vi "340 Read and Compressor auto control(SubVI).vi"(11 "Instrument":T2={"limit"={"Field limit"=0.0, "Field rate limit"=0.0, "Temp limit"=0.0, "Temp low limit"=0.0, "Temp rate limit "=0.0}, "genarl"={"行数"=refnum, "编辑列表框？"=refnum, "列表框"=refnum, "camg 振荡状态"=refnum, "Aborting"=refnum, "数据文件"=refnum, "warning"=refnum, "vi路径"="", "Instrument Type"=enum."PPMS-Rotate"}, "cmag"={"TM620"="TCPIP0::192.168.1.5::4266::SOCKET", "M24C Resource"="GPIB0::24::INSTR", "4G supply"="", "Temp Status 24C"=refnum, "Temp"=refnum, "9T信号"=refnum, "4g supply status"=refnum, "in-plane"="", "out-plane"="", "in-plane signal"=FALSE, "out-plane signal"=FALSE, "in plane 信号"=refnum, "pzt volt"=refnum, "camg Rate"=refnum}, "lengtou2"={"750 visa"="", "750 rotate"="", "semaphore 340"=refnum, "semaphore 750"=refnum, "750 field status"=refnum, "Input (0:A) 340"=0, "340 Resource"="GPIB0::14::INSTR", "340 Status"=refnum, "Input (0:B) 340"=1, "Loop (0: 1)"=0, "Loop (1: 1)"=0, "TCP master instance"=refnum}, "lengtou"={"TCP master instance"=refnum, "335 Status"=refnum, "335 Resource "="GPIB0::24::INSTR", "Input (0:A) 335"=0, "Input (0:B) 335"=1, "Heater Output (1:1) 335"=1, "semaphore 335"=refnum}, "325 for test"={"quantum design"=refnum, "semaphore 325"=refnum, "325 Resource "="GPIB0::13::INSTR", "Input (0:A) 325"=0, "Heater Output (1:1) 325"=1, "325 Status"=refnum}} {"325 for test"."Heater Output (1:1) 325" items=["1"=1, "2"=2]; "325 for test"."Input (0:A) 325" items=["A", "B"]; "lengtou"."Heater Output (1:1) 335" items=["1"=1, "2"=2]; "lengtou"."Input (0:B) 335" items=["A", "B"]; "lengtou"."Input (0:A) 335" items=["A", "B"]; "lengtou2"."Loop (1: 1)" items=["1", "2"]; "lengtou2"."Loop (0: 1)" items=["1", "2"]; "lengtou2"."Input (0:B) 340" items=["A", "B", "C", "D"]; "lengtou2"."Input (0:A) 340" items=["A", "B", "C", "D"]}) -> (2 "Output Field (Gs)":dbl, 3 "output":T7 {"?" items=["Unknow", "Stable", "Following Warm", "Following Cold", "Unfollowing"]; "?" items=["Unknow", "Stable", "Following Warm", "Following Cold", "Unfollowing"]}, 9 "field status 2":T1=enum."Stable")   [LabVIEW 2019, in "Get value.lvlib"]
uses:
  Get value.lvlib
  ctl/335 state.ctl
  ctl/Instrument.ctl
  <vilib>/NI/Modbus Library/API/Master/Modbus Master.lvclass
  ctl/limit.ctl
  ctl/warning.ctl
  ctl/Instrument Type.ctl
  ctl/9T mag field stauts.ctl
  C:/Users/fuyang/Desktop/postdoctor/labview/labview-measure/lib/QDInstrument.dll
  lib/QDInstrument.dll
  lib/Lake Shore 340/Lake Shore Cryotronics 340.lvlib
  User lib.lvlib
panel:
  out "下拉列表 2":T6=2 items=["Unknow", "Stable", "Following Warm", "Following Cold", "Unfollowing"]
  out "下拉列表":T6=2 items=["Unknow", "Stable", "Following Warm", "Following Cold", "Unfollowing"]
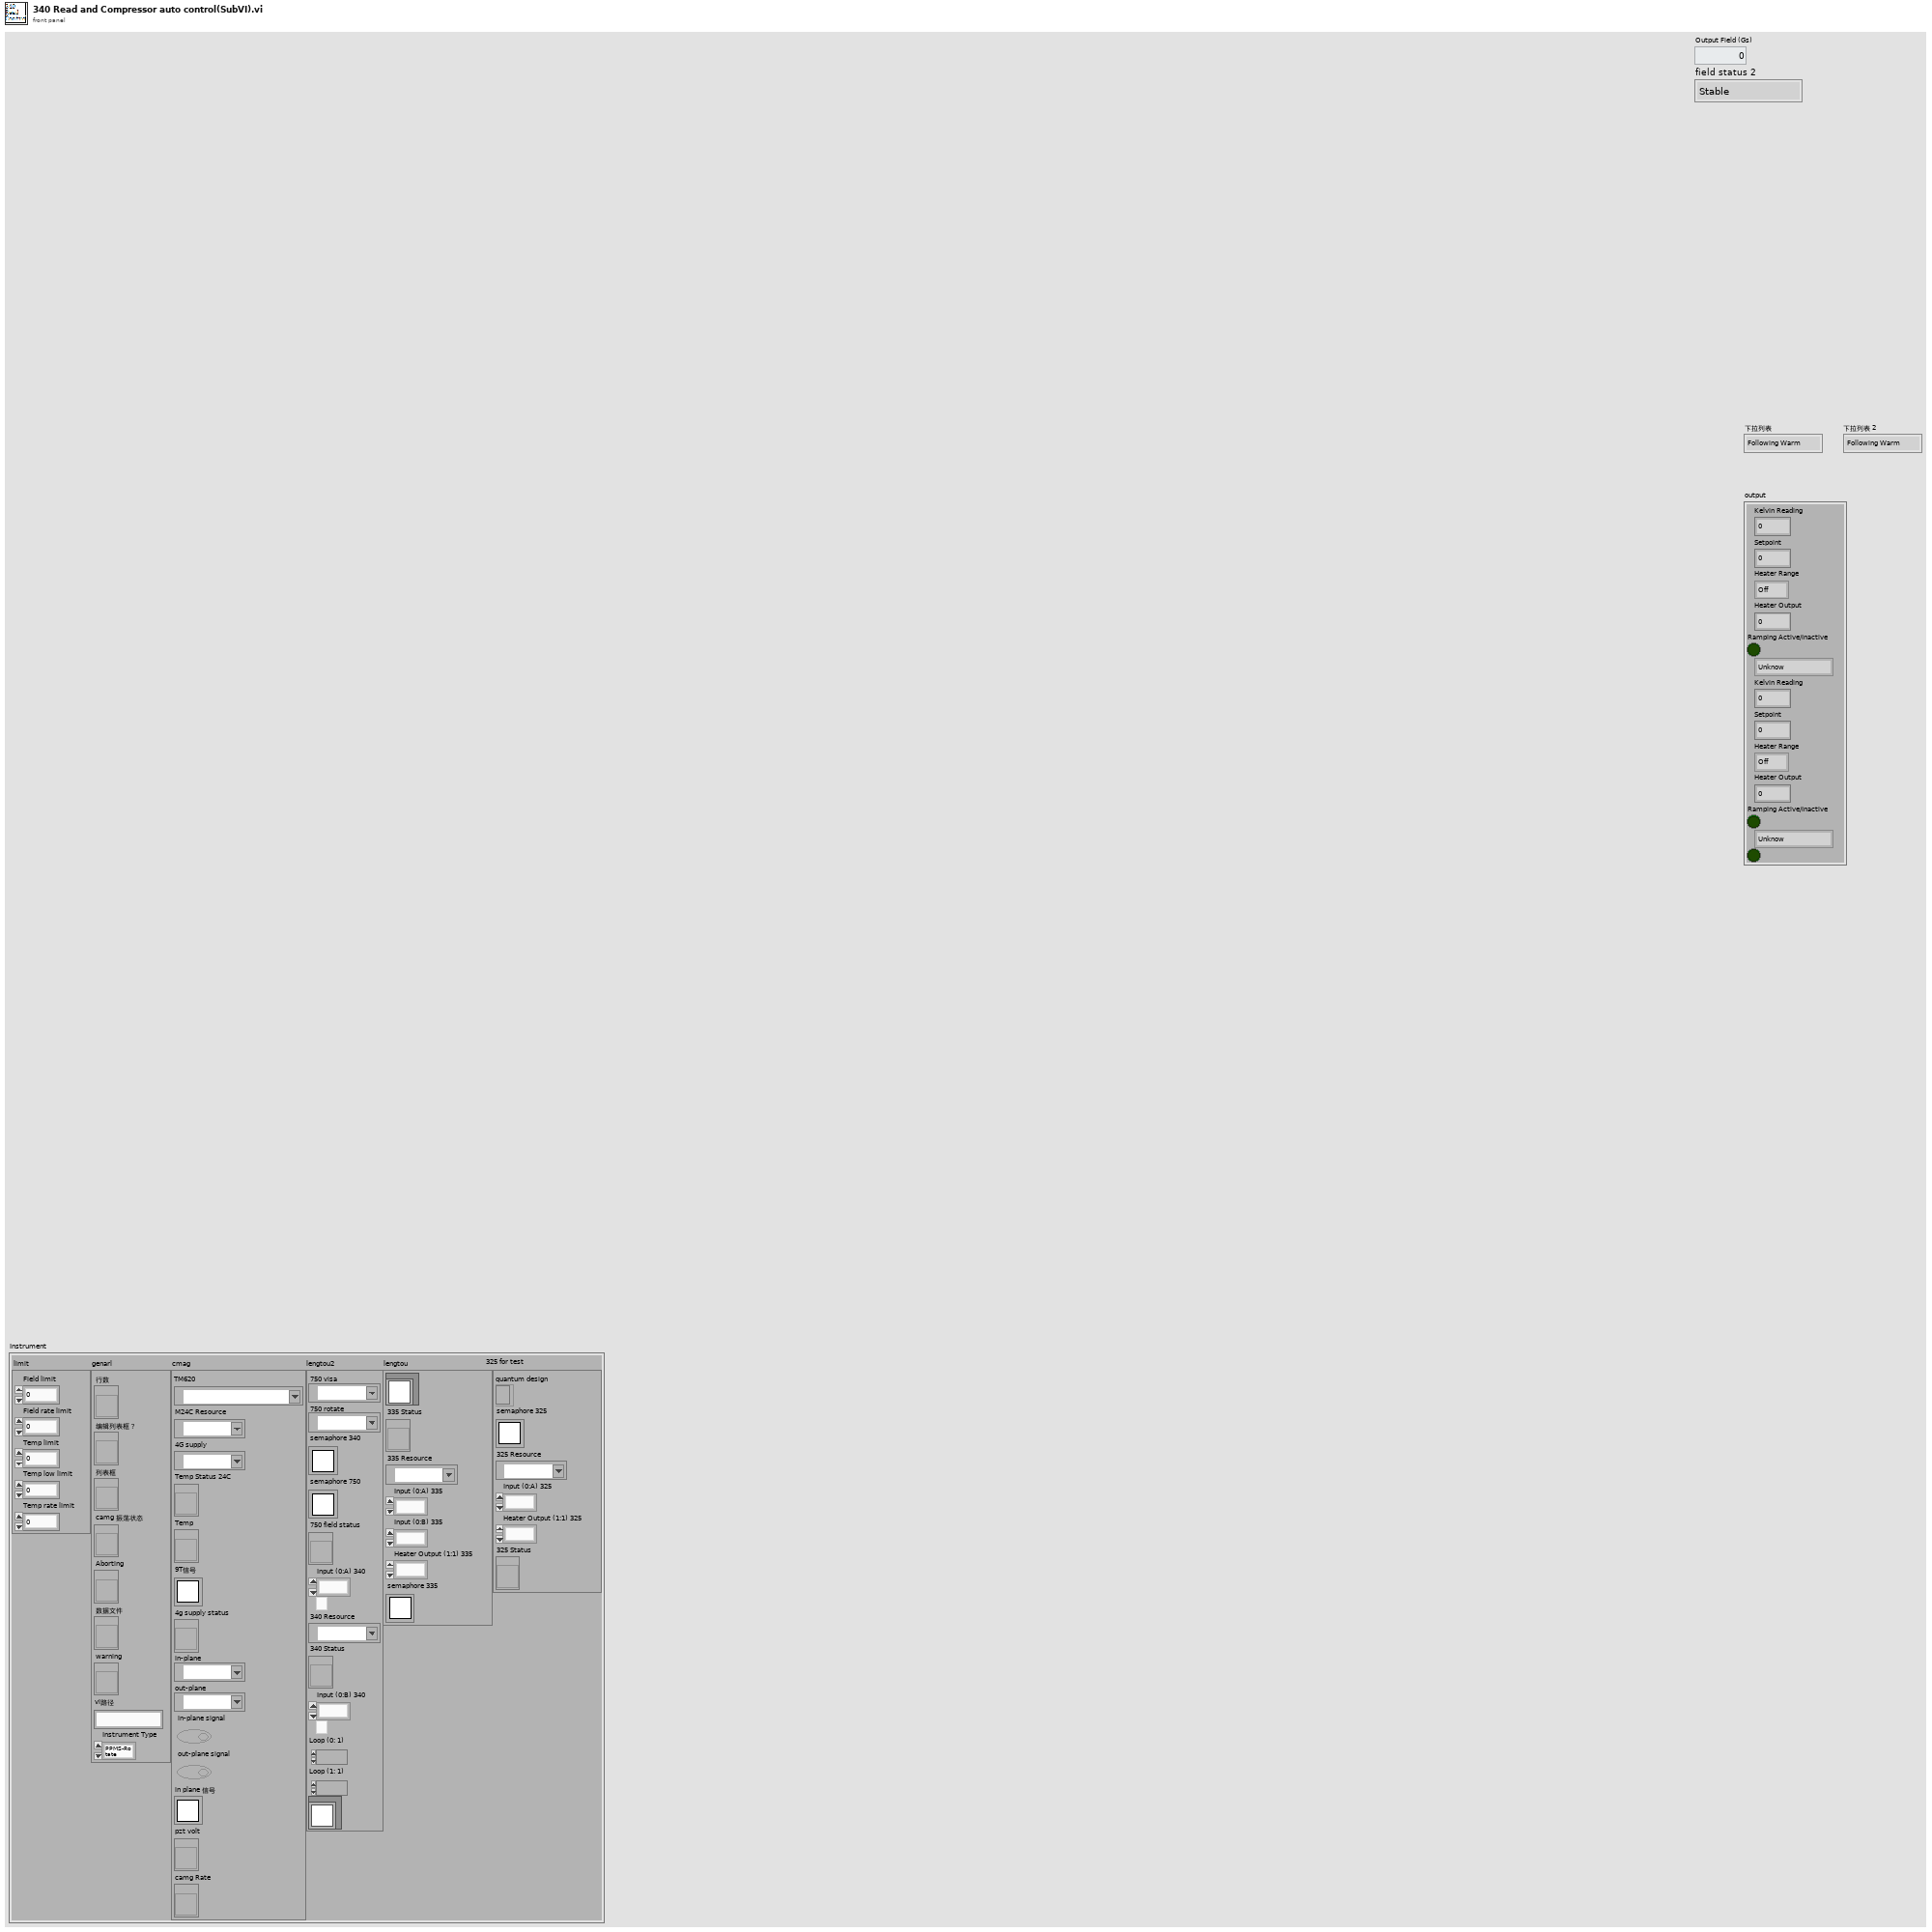
[diagram p1: front panel]
types:
  T1 = typedef "9T mag field stauts.ctl" = enum16{"unknow", "Stable", "Sweep up", "Sweep down", "Sweep to zero", "Pause"}
  T2 = typedef "Instrument.ctl" = cluster{"limit":T3, "genarl":cluster{"行数":refnum<vi>, "编辑列表框？":refnum<vi>, "列表框":refnum<vi>, "camg 振荡状态":refnum<vi>, "Aborting":refnum<vi>, "数据文件":refnum<vi>, "warning":refnum<vi>, "vi路径":string, "Instrument Type":T4}, "cmag":cluster{"TM620":refnum<visa-resource-name>, "M24C Resource":refnum<visa-resource-name>, "4G supply":refnum<visa-resource-name>, "Temp Status 24C":refnum<vi>, "Temp":refnum<vi>, "9T信号":T5, "4g supply status":refnum<vi>, "in-plane":refnum<visa-resource-name>, "out-plane":refnum<visa-resource-name>, "in-plane signal":bool, "out-plane signal":bool, "in plane 信号":T5, "pzt volt":refnum<vi>, "camg Rate":refnum<vi>}, "lengtou2":cluster{"750 visa":refnum<visa-resource-name>, "750 rotate":refnum<visa-resource-name>, "semaphore 340":T5, "semaphore 750":T5, "750 field status":refnum<vi>, "Input (0:A) 340":u16, "340 Resource":refnum<visa-resource-name>, "340 Status":refnum<vi>, "Input (0:B) 340":u16, "Loop (0: 1)":u16, "Loop (1: 1)":u16, "TCP master instance":refnum<class "Modbus Master.lvclass">}, "lengtou":cluster{"TCP master instance":refnum<class "Modbus Master.lvclass">, "335 Status":refnum<vi>, "335 Resource ":refnum<visa-resource-name>, "Input (0:A) 335":u16, "Input (0:B) 335":u16, "Heater Output (1:1) 335":u16, "semaphore 335":T5}, "325 for test":cluster{"quantum design":refnum<k24>, "semaphore 325":T5, "325 Resource ":refnum<visa-resource-name>, "Input (0:A) 325":u16, "Heater Output (1:1) 325":u16, "325 Status":refnum<vi>}}
  T3 = typedef "limit.ctl" = cluster{"Field limit":dbl, "Field rate limit":dbl, "Temp limit":dbl, "Temp low limit":dbl, "Temp rate limit ":dbl}
  T4 = typedef "Instrument Type.ctl" = enum16{"PPMS", "VersaLab", "DynaCool", "SVSM", "PPMS-Rotate", "Lakeshore335", "2T cmag", "9T mag old", "9T cmag", "9T cmag DAC", "9T cmag rotate", "test"}
  T5 = typedef "Semaphore RefNum" = refnum<k1>
  T6 = typedef "335 state.ctl" = u16
  T7 = cluster{"Kelvin Reading":dbl, "Setpoint":dbl, "Heater Range":enum16{"Off", "1", "2", "3", "4", "5"}, "Heater Output":dbl, "Ramping Active/Inactive":bool, T6, "Kelvin Reading":dbl, "Setpoint":dbl, "Heater Range":enum16{"Off", "1", "2", "3", "4", "5"}, "Heater Output":dbl, "Ramping Active/Inactive":bool, T6, bool}
  T8 = cluster{"Kelvin Reading":dbl, "Setpoint":dbl, "Heater Range 340-Loop2":i32, "Output Value":dbl, "Ramping Active/Inactive":bool, T6, "Kelvin Reading":dbl, "Setpoint":dbl, "Heater Range":enum16{"Off", "1", "2", "3", "4", "5"}, "Heater Output":dbl, "Ramping Active/Inactive":bool, T6, bool}
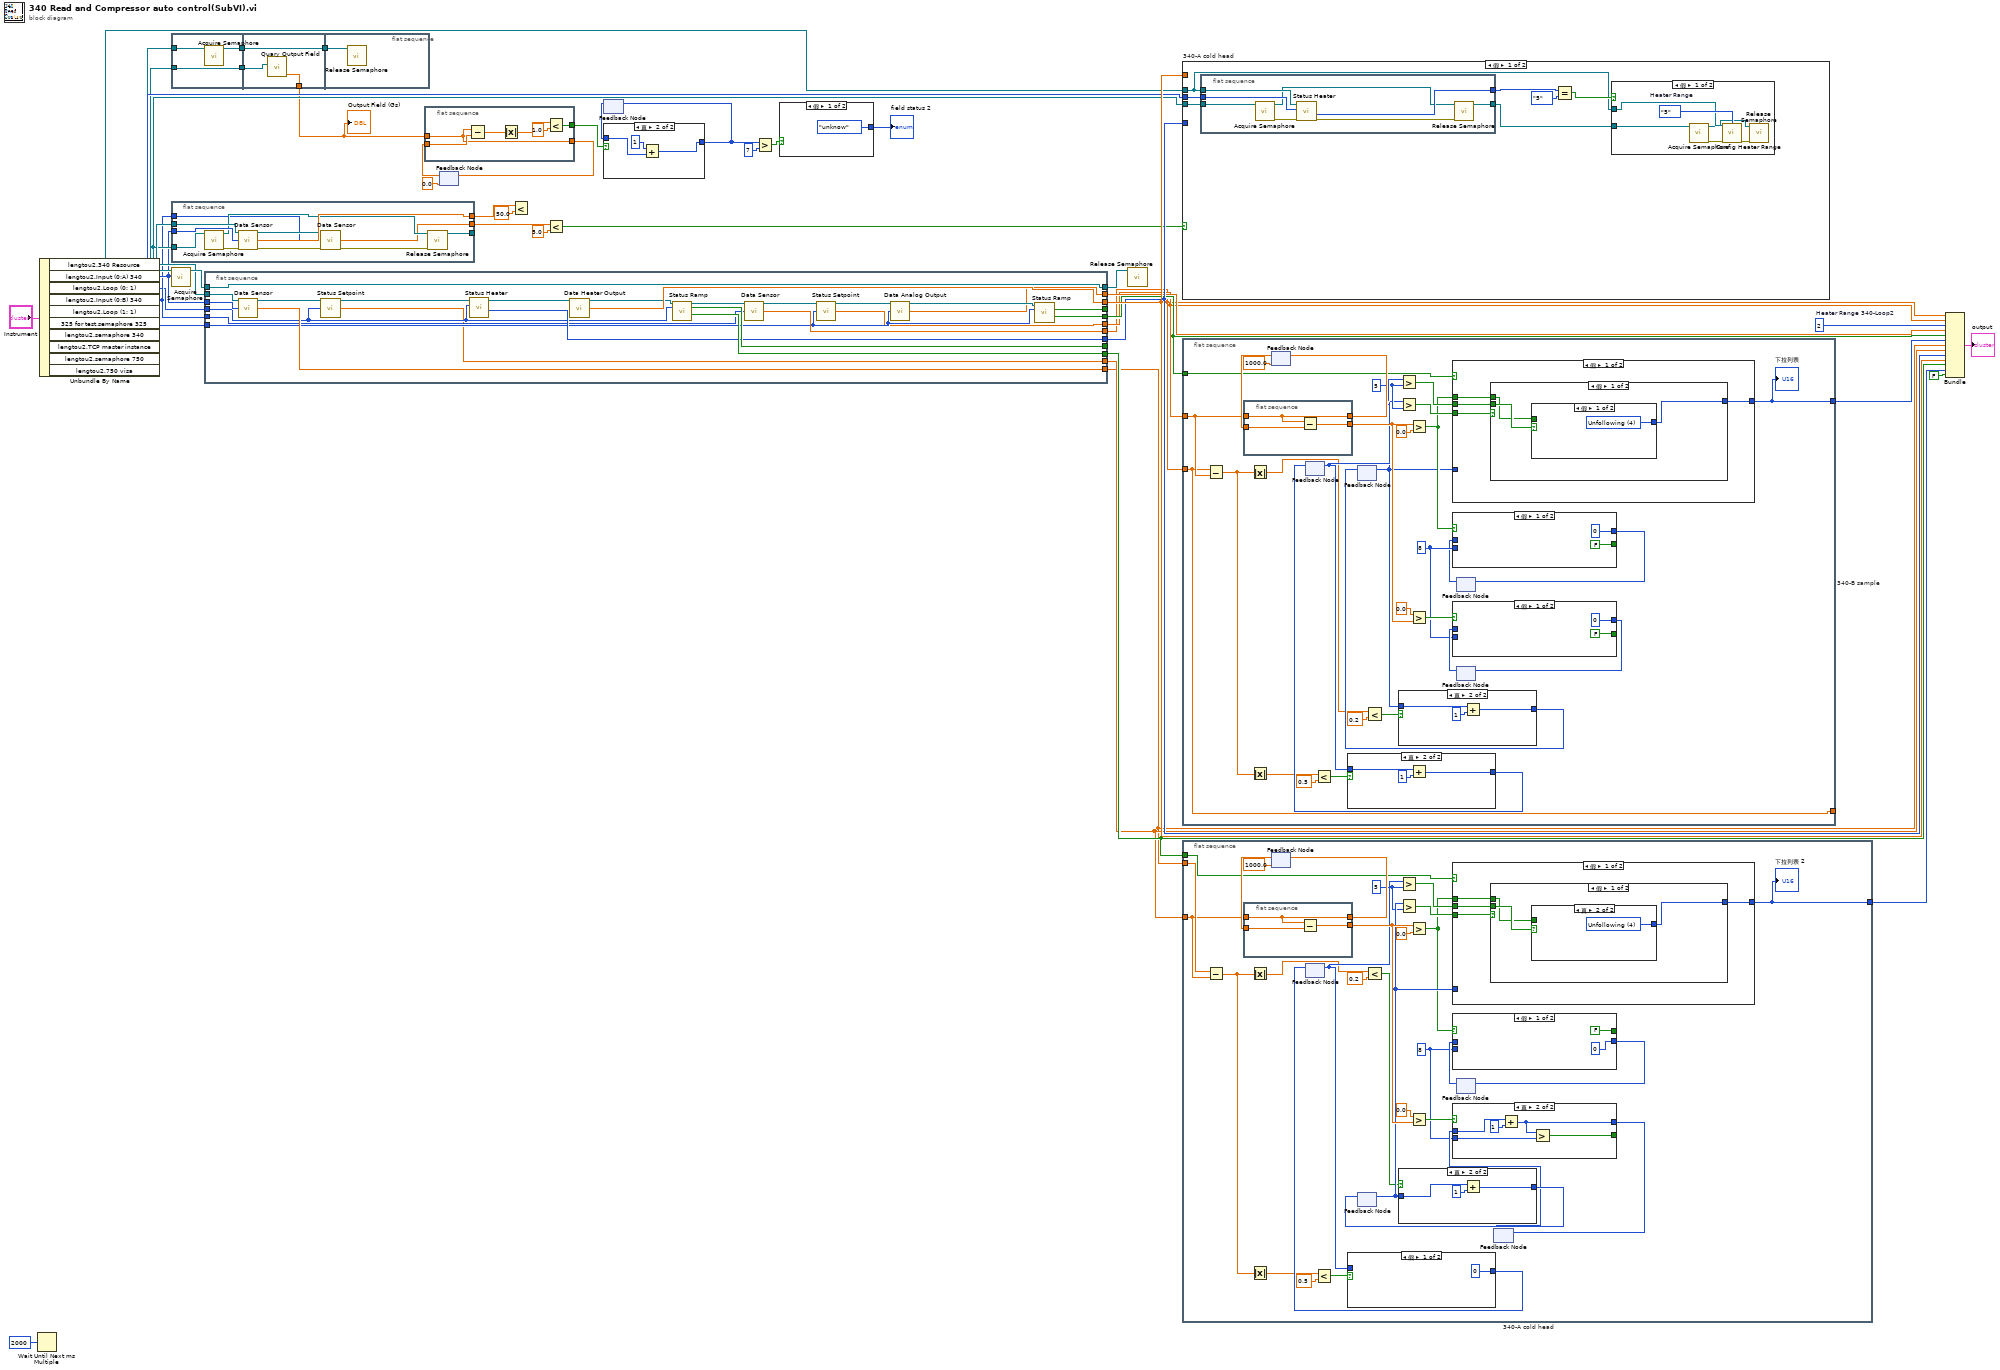
[diagram p0: block diagram]
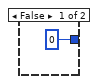
[diagram p2: hidden frame]
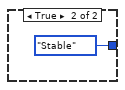
[diagram p3: hidden frame]
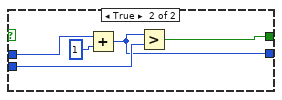
[diagram p4: hidden frame]
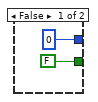
[diagram p5: hidden frame]
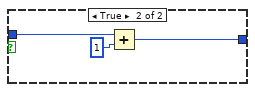
[diagram p6: hidden frame]
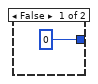
[diagram p7: hidden frame]
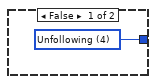
[diagram p8: hidden frame]
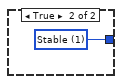
[diagram p9: hidden frame]
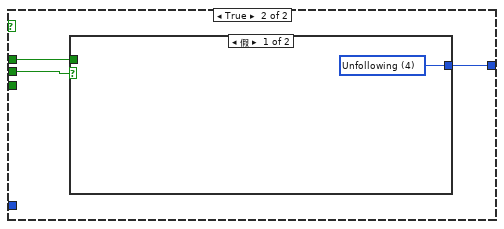
[diagram p10: hidden frame]
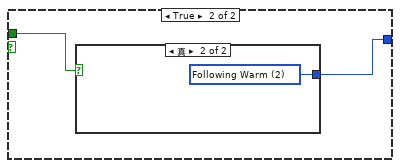
[diagram p11: hidden frame]
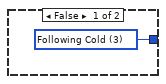
[diagram p12: hidden frame]
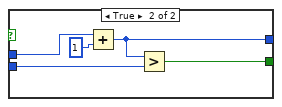
[diagram p13: hidden frame]
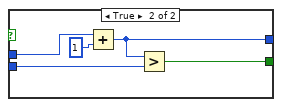
[diagram p14: hidden frame]
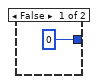
[diagram p15: hidden frame]
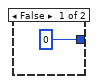
[diagram p16: hidden frame]
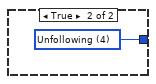
[diagram p17: hidden frame]
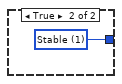
[diagram p18: hidden frame]
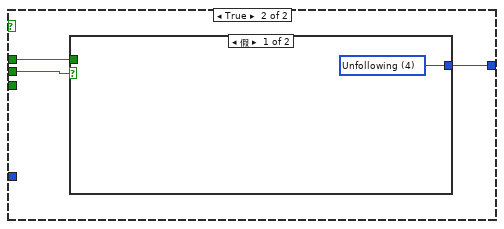
[diagram p19: hidden frame]
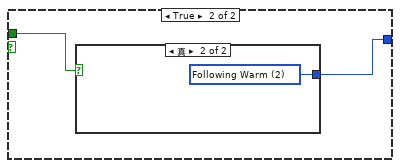
[diagram p20: hidden frame]
diagram:
  w22 = 2  # Heater Range 340-Loop2
  n1 = Wait Until Next ms Multiple(millisecond multiple=u32 2000) -> ()  [unwired: 1 out]
  n2 = Unbundle By Name("Instrument") -> ("lengtou2.340 Resource"=w31:refnum<visa-resource-name>, "lengtou2.Input (0:A) 340"=w28:u16, "lengtou2.Loop (0: 1)"=w24:u16, "lengtou2.Input (0:B) 340"=w27:u16, "lengtou2.Loop (1: 1)"=w23:u16, "lengtou2.semaphore 340"=w29:T5, "lengtou2.semaphore 750"=w17:T5, "lengtou2.750 visa"=w19:refnum<visa-resource-name>)  [unwired: 2 out]
  n3 = flat-sequence {
    tunnel: w19 -> [w47]
    tunnel: [w47] -> w18
    tunnel: w17 -> [w45]
    tunnel: [w46] -> w16
    tunnel: w18 -> [w50]
    tunnel: w16 -> [w49]
    tunnel: [w49] -> w15
    tunnel: [w48] -> w14
    tunnel: w15 -> [w51]
    frame #0 {
      n4 = call <vilib>:"Acquire Semaphore.vi"("semaphore"=w45) -> ("semaphore out"=w46:T5)  [unwired: 4 in, 2 out]
    }
    frame #1 {
      n5 = call "Quary Output Field.vi"("VISA resource name"=w50) -> ("Output Field (Gs)"=w48:dbl)  [unwired: 8 in, 2 out]
    }
    frame #2 {
      n6 = call <vilib>:"Release Semaphore.vi"("semaphore"=w51) -> ()  [unwired: 5 in, 2 out]
    }
  }
  n7 = flat-sequence {
    tunnel: [w63] -> w32
    tunnel: w31 -> [w62]
    tunnel: w28 -> [w61]
    tunnel: w29 -> [w60]
    tunnel: [w57] -> _
    tunnel: w27 -> [w53]
    tunnel: [w52] -> w30
    frame #0 {
      n8 = call <vilib>:"Acquire Semaphore.vi"("semaphore"=w60) -> ("error out"=w59:errorcluster, "semaphore out"=w58:T5)  [unwired: 4 in, 1 out]
      n9 = call "Data Sensor.vi"("VISA resource name"=w62, "Input (0: A)"=w61, "error in (no error)"=w59) -> ("VISA resource name out"=w54:refnum<visa-resource-name>, "Kelvin Reading"=w63:dbl, "error out"=w56:errorcluster)  [unwired: 8 in, 2 out]
      n10 = call "Data Sensor.vi"("VISA resource name"=w54, "Input (0: A)"=w53, "error in (no error)"=w56) -> ("Kelvin Reading"=w52:dbl, "error out"=w55:errorcluster)  [unwired: 8 in, 3 out]
      n11 = call <vilib>:"Release Semaphore.vi"("error in (no error)"=w55, "semaphore"=w58) -> ("semaphore out"=w57:T5)  [unwired: 4 in, 1 out]
    }
  }
  n12 = call <vilib>:"Acquire Semaphore.vi"("semaphore"=w29) -> ("semaphore out"=w42:T5)  [unwired: 4 in, 2 out]
  n13 = flat-sequence {
    tunnel: [w64] -> w4
    tunnel: w31 -> [w87]
    tunnel: w42 -> [w88]
    tunnel: [w88] -> w43
    tunnel: w28 -> [w77]
    tunnel: [w86] -> w37
    tunnel: [w85] -> w2
    tunnel: [w83] -> _
    tunnel: [w82] -> w41
    tunnel: w24 -> [w68]
    tunnel: [w78] -> w38
    tunnel: [w76] -> w1
    tunnel: w27 -> [w74]
    tunnel: [w65] -> w3
    tunnel: [w71] -> w25
    tunnel: [w70] -> _
    tunnel: [w69] -> w26
    tunnel: w23 -> [w67]
    frame #0 {
      n14 = call "Data Sensor.vi"("VISA resource name"=w87, "Input (0: A)"=w77) -> ("VISA resource name out"=w84:refnum<visa-resource-name>, "Kelvin Reading"=w85:dbl)  [unwired: 9 in, 3 out]
      n15 = call "Status Setpoint.vi"("VISA resource name"=w84, "Loop (0: 1)"=w68) -> ("VISA resource name out"=w80:refnum<visa-resource-name>, "Setpoint"=w64:dbl)  [unwired: 11 in, 1 out]
      n16 = call "Status Heater.vi"("Loop"=w68, "VISA resource name"=w80) -> ("Heater Range"=w78:enum16{"Off", "1", "2", "3", "4", "5"}, "VISA resource name out"=w79:refnum<visa-resource-name>)  [unwired: 7 in, 1 out]
      n17 = call "Data Heater Output.vi"("VISA resource name"=w79) -> ("VISA resource name out"=w81:refnum<visa-resource-name>, "Heater Output"=w82:dbl)  [unwired: 12 in, 1 out]
      n18 = call "Status Ramp.vi"("VISA resource name"=w81, "Loop (0: 1)"=w68) -> ("VISA resource name out"=w75:refnum<visa-resource-name>, "Ramping On/Off"=w83:bool, "Ramping Active/Inactive"=w86:bool)  [unwired: 9 in, 2 out]
      n19 = call "Data Sensor.vi"("VISA resource name"=w75, "Input (0: A)"=w74) -> ("VISA resource name out"=w73:refnum<visa-resource-name>, "Kelvin Reading"=w76:dbl)  [unwired: 9 in, 3 out]
      n20 = call "Status Setpoint.vi"("VISA resource name"=w73, "Loop (0: 1)"=w67) -> ("VISA resource name out"=w66:refnum<visa-resource-name>, "Setpoint"=w65:dbl)  [unwired: 11 in, 1 out]
      n21 = call "Data Analog Output.vi"("VISA resource name"=w66, "Analog Output (0: 1)"=w67) -> ("VISA resource name out"=w72:refnum<visa-resource-name>, "Output Value"=w71:dbl)  [unwired: 11 in, 1 out]
      n22 = call "Status Ramp.vi"("VISA resource name"=w72, "Loop (0: 1)"=w67) -> ("Ramping On/Off"=w70:bool, "Ramping Active/Inactive"=w69:bool)  [unwired: 9 in, 3 out]
    }
  }
  n23 = flat-sequence {
    tunnel: w14 -> [w90]
    tunnel: w12 -> [w91]
    tunnel: [w90] -> w13
    tunnel: [w92] -> w11
    frame #0 {
      n24 = Subtract(x=w90, y=w91) -> (x-y=w89:dbl)
      n25 = Absolute Value(x=w89) -> (abs(x)=w94:dbl)
      n26 = Less?(x=w94, y=1.0) -> (x < y?=w92:bool)
    }
  }
  n27 = feedback #1(0.0) -> (w12:dbl)
  n28 = feedback-in #1(w13) -> ()
  n29 = Less?(x=w32, y=50.0) -> ()  [unwired: 1 out]
  n30 = Less?(x=w30, y=5.0) -> (x < y?=w34:bool)
  n31 = feedback #2() -> (w10:i32)  [unwired: 1 in]
  n32 = case shown="真" w11 {
    tunnel: [0 w96] -> w9
    tunnel: w10 -> [_ w98]
    frame False {
    }
    frame True {
      n33 = Add(x=1, y=w98) -> (x+y=w96:i32)
    }
  }
  n34 = feedback-in #2(w9) -> ()
  n35 = Greater?(x=w9, y=7) -> (0:w7:bool)
  n36 = case shown="假" w7 {
    tunnel: [9T_mag_field_stauts."unknow" ("field stauts") 9T_mag_field_stauts."Stable" ("field stauts")] -> w5
    frame False {
    }
    frame True {
    }
  }
  "field status 2" <- w5
  n37 = call <vilib>:"Release Semaphore.vi"("semaphore"=w43) -> ()  [unwired: 5 in, 2 out]
  n38 = case "340-A cold head" shown="假" w34 {
    tunnel: w41 -> [_ w133]
    tunnel: w31 -> [w103 w130]
    tunnel: w29 -> [w101 w129]
    tunnel: w38 -> [_ w122]
    tunnel: w23 -> [w107 _]
    frame False {
      n39 = flat-sequence {
        tunnel: w107 -> [w115]
        tunnel: [w114] -> w106
        tunnel: w103 -> [w113]
        tunnel: w101 -> [w109]
        tunnel: [w108] -> w102
        frame #0 {
          n40 = call <vilib>:"Acquire Semaphore.vi"("semaphore"=w109) -> ("error out"=w111:errorcluster, "semaphore out"=w110:T5)  [unwired: 4 in, 1 out]
          n41 = call "Status Heater.vi"("error in (no error)"=w111, "Loop"=w115, "VISA resource name"=w113) -> ("error out"=w112:errorcluster, "Heater Range"=w114:enum16{"Off", "1", "2", "3", "4", "5"})  [unwired: 6 in, 1 out]
          n42 = call <vilib>:"Release Semaphore.vi"("error in (no error)"=w112, "semaphore"=w110) -> ("semaphore out"=w108:T5)  [unwired: 4 in, 1 out]
        }
      }
      n43 = Equal?(x=w106, y=enum16{"Off", "1", "2", "3", "4", "5"}."5" ("Heater Range")) -> (x = y?=w104:bool)
      n44 = case shown="假" w104 {
        tunnel: w103 -> [w120 _]
        tunnel: w102 -> [w118 _]
        frame False {
          w121 = enum16{"Off", "1", "2", "3", "4", "5"}."5"  # Heater Range
          n45 = call <vilib>:"Acquire Semaphore.vi"("semaphore"=w118) -> ("error out"=w117:errorcluster, "semaphore out"=w116:T5)  [unwired: 4 in, 1 out]
          n46 = call "Config Heater Range.vi"("VISA resource name"=w120, "Heater Range (0: Off)"=w121, "error in (no error)"=w117) -> ("error out"=w119:errorcluster)  [unwired: 11 in, 1 out]
          n47 = call <vilib>:"Release Semaphore.vi"("error in (no error)"=w119, "semaphore"=w116) -> ()  [unwired: 4 in, 2 out]
        }
        frame True {
        }
      }
    }
    frame True {
      n48 = Less?(x=w133, y=5.0) -> (x < y?=w124:bool)
      n49 = Greater?(x=w133, y=80.0) -> (0:w131:bool)
      n50 = feedback #3(0) -> (w125:i32)
      n51 = Greater?(x=w125, y=3) -> (0:w127:bool)
      n52 = case shown="真" w127 {
        tunnel: w131 -> [_ w144]
        tunnel: w130 -> [_ w143]
        tunnel: w129 -> [_ w142]
        tunnel: [w135 w141] -> w126
        tunnel: w125 -> [w137 w140]
        tunnel: w124 -> [_ w139]
        tunnel: w122 -> [_ w138]
        frame False {
          n53 = Add(x=1, y=w137) -> (x+y=w135:i32)
        }
        frame True {
          n54 = case shown="假" w144 {
            tunnel: w143 -> [w150 w201]
            tunnel: w142 -> [w147 w200]
            tunnel: [w149 w199] -> w141
            tunnel: w140 -> [w148 w198]
            tunnel: w139 -> [w146 _]
            tunnel: w138 -> [w145 w197]
            frame False {
              n55 = case shown="真" w146 {
                tunnel: w150 -> [_ w157]
                tunnel: [w151 w158] -> w149
                tunnel: w148 -> [w153 w155]
                tunnel: w147 -> [_ w156]
                tunnel: w145 -> [_ w154]
                frame False {
                  n56 = Add(x=1, y=w153) -> (x+y=w151:i32)
                }
                frame True {
                  n57 = case shown="\"5\"" w154 {
                    tunnel: w157 -> [w161 w167 w174 w182 _ w191]
                    tunnel: w156 -> [w160 w166 w173 w181 _ w193]
                    tunnel: [0 0 0 0 w187 0] -> w158
                    tunnel: w155 -> [_ _ _ _ w188 _]
                    frame "Off" {
                      w162 = enum16{"Off", "1", "2", "3", "4", "5"}."4"  # Heater Range
                      n58 = call <vilib>:"Acquire Semaphore.vi"("semaphore"=w160) -> ("error out"=w165:errorcluster, "semaphore out"=w163:T5)  [unwired: 4 in, 1 out]
                      n59 = call "Config Heater Range.vi"("VISA resource name"=w161, "Heater Range (0: Off)"=w162, "error in (no error)"=w165) -> ("error out"=w164:errorcluster)  [unwired: 11 in, 1 out]
                      n60 = call <vilib>:"Release Semaphore.vi"("error in (no error)"=w164, "semaphore"=w163) -> ()  [unwired: 4 in, 2 out]
                    }
                    frame "1", Default {
                      w169 = enum16{"Off", "1", "2", "3", "4", "5"}."4"  # Heater Range
                      n61 = call <vilib>:"Acquire Semaphore.vi"("semaphore"=w166) -> ("error out"=w172:errorcluster, "semaphore out"=w170:T5)  [unwired: 4 in, 1 out]
                      n62 = call "Config Heater Range.vi"("VISA resource name"=w167, "Heater Range (0: Off)"=w169, "error in (no error)"=w172) -> ("error out"=w171:errorcluster)  [unwired: 11 in, 1 out]
                      n63 = call <vilib>:"Release Semaphore.vi"("error in (no error)"=w171, "semaphore"=w170) -> ()  [unwired: 4 in, 2 out]
                    }
                    frame "2" {
                      w175 = enum16{"Off", "1", "2", "3", "4", "5"}."4"  # Heater Range
                      n64 = call <vilib>:"Acquire Semaphore.vi"("semaphore"=w173) -> ("error out"=w178:errorcluster, "semaphore out"=w176:T5)  [unwired: 4 in, 1 out]
                      n65 = call "Config Heater Range.vi"("VISA resource name"=w174, "Heater Range (0: Off)"=w175, "error in (no error)"=w178) -> ("error out"=w177:errorcluster)  [unwired: 11 in, 1 out]
                      n66 = call <vilib>:"Release Semaphore.vi"("error in (no error)"=w177, "semaphore"=w176) -> ()  [unwired: 4 in, 2 out]
                    }
                    frame "3" {
                      w183 = enum16{"Off", "1", "2", "3", "4", "5"}."4"  # Heater Range
                      n67 = call <vilib>:"Acquire Semaphore.vi"("semaphore"=w181) -> ("error out"=w186:errorcluster, "semaphore out"=w184:T5)  [unwired: 4 in, 1 out]
                      n68 = call "Config Heater Range.vi"("VISA resource name"=w182, "Heater Range (0: Off)"=w183, "error in (no error)"=w186) -> ("error out"=w185:errorcluster)  [unwired: 11 in, 1 out]
                      n69 = call <vilib>:"Release Semaphore.vi"("error in (no error)"=w185, "semaphore"=w184) -> ()  [unwired: 4 in, 2 out]
                    }
                    frame "4" {
                      n70 = Add(x=1, y=w188) -> (x+y=w187:i32)
                    }
                    frame "5" {
                      w192 = enum16{"Off", "1", "2", "3", "4", "5"}."4"  # Heater Range
                      n71 = call <vilib>:"Acquire Semaphore.vi"("semaphore"=w193) -> ("error out"=w196:errorcluster, "semaphore out"=w194:T5)  [unwired: 4 in, 1 out]
                      n72 = call "Config Heater Range.vi"("VISA resource name"=w191, "Heater Range (0: Off)"=w192, "error in (no error)"=w196) -> ("error out"=w195:errorcluster)  [unwired: 11 in, 1 out]
                      n73 = call <vilib>:"Release Semaphore.vi"("error in (no error)"=w195, "semaphore"=w194) -> ()  [unwired: 4 in, 2 out]
                    }
                  }
                }
              }
            }
            frame True {
              n74 = case shown="\"5\"" w197 {
                tunnel: w201 -> [w203 w210 w217 w225 w232 _]
                tunnel: w200 -> [w202 w212 w216 w224 w231 _]
                tunnel: [0 0 0 0 0 w237] -> w199
                tunnel: w198 -> [_ _ _ _ _ w238]
                frame "Off" {
                  w205 = enum16{"Off", "1", "2", "3", "4", "5"}."4"  # Heater Range
                  n75 = call <vilib>:"Acquire Semaphore.vi"("semaphore"=w202) -> ("error out"=w208:errorcluster, "semaphore out"=w206:T5)  [unwired: 4 in, 1 out]
                  n76 = call "Config Heater Range.vi"("VISA resource name"=w203, "Heater Range (0: Off)"=w205, "error in (no error)"=w208) -> ("error out"=w207:errorcluster)  [unwired: 11 in, 1 out]
                  n77 = call <vilib>:"Release Semaphore.vi"("error in (no error)"=w207, "semaphore"=w206) -> ()  [unwired: 4 in, 2 out]
                }
                frame "1", Default {
                  w211 = enum16{"Off", "1", "2", "3", "4", "5"}."4"  # Heater Range
                  n78 = call <vilib>:"Acquire Semaphore.vi"("semaphore"=w212) -> ("error out"=w215:errorcluster, "semaphore out"=w213:T5)  [unwired: 4 in, 1 out]
                  n79 = call "Config Heater Range.vi"("VISA resource name"=w210, "Heater Range (0: Off)"=w211, "error in (no error)"=w215) -> ("error out"=w214:errorcluster)  [unwired: 11 in, 1 out]
                  n80 = call <vilib>:"Release Semaphore.vi"("error in (no error)"=w214, "semaphore"=w213) -> ()  [unwired: 4 in, 2 out]
                }
                frame "2" {
                  w218 = enum16{"Off", "1", "2", "3", "4", "5"}."4"  # Heater Range
                  n81 = call <vilib>:"Acquire Semaphore.vi"("semaphore"=w216) -> ("error out"=w221:errorcluster, "semaphore out"=w219:T5)  [unwired: 4 in, 1 out]
                  n82 = call "Config Heater Range.vi"("VISA resource name"=w217, "Heater Range (0: Off)"=w218, "error in (no error)"=w221) -> ("error out"=w220:errorcluster)  [unwired: 11 in, 1 out]
                  n83 = call <vilib>:"Release Semaphore.vi"("error in (no error)"=w220, "semaphore"=w219) -> ()  [unwired: 4 in, 2 out]
                }
                frame "3" {
                  w226 = enum16{"Off", "1", "2", "3", "4", "5"}."4"  # Heater Range
                  n84 = call <vilib>:"Acquire Semaphore.vi"("semaphore"=w224) -> ("error out"=w229:errorcluster, "semaphore out"=w227:T5)  [unwired: 4 in, 1 out]
                  n85 = call "Config Heater Range.vi"("VISA resource name"=w225, "Heater Range (0: Off)"=w226, "error in (no error)"=w229) -> ("error out"=w228:errorcluster)  [unwired: 11 in, 1 out]
                  n86 = call <vilib>:"Release Semaphore.vi"("error in (no error)"=w228, "semaphore"=w227) -> ()  [unwired: 4 in, 2 out]
                }
                frame "4" {
                  w233 = enum16{"Off", "1", "2", "3", "4", "5"}."5"  # Heater Range
                  n87 = call <vilib>:"Acquire Semaphore.vi"("semaphore"=w231) -> ("error out"=w236:errorcluster, "semaphore out"=w234:T5)  [unwired: 4 in, 1 out]
                  n88 = call "Config Heater Range.vi"("VISA resource name"=w232, "Heater Range (0: Off)"=w233, "error in (no error)"=w236) -> ("error out"=w235:errorcluster)  [unwired: 11 in, 1 out]
                  n89 = call <vilib>:"Release Semaphore.vi"("error in (no error)"=w235, "semaphore"=w234) -> ()  [unwired: 4 in, 2 out]
                }
                frame "5" {
                  n90 = Add(x=1, y=w238) -> (x+y=w237:i32)
                }
              }
            }
          }
        }
      }
      n91 = feedback-in #3(w126) -> ()
    }
  }
  n92 = flat-sequence "340-B sample" {
    tunnel: w1 -> [w242]
    tunnel: w3 -> [w245]
    tunnel: w26 -> [w244]
    tunnel: [w243] -> w39
    tunnel: [w242] -> _
    frame #0 {
      w246 = 8 ("y")
      w259 = 5 ("y")
      n93 = Subtract(x=w242, y=w245) -> (x-y=w257:dbl)
      n94 = flat-sequence {
        tunnel: w245 -> [w287]
        tunnel: [w287] -> w265
        tunnel: w266 -> [w286]
        tunnel: [w285] -> w270
        frame #0 {
          n95 = Subtract(x=w287, y=w286) -> (x-y=w285:dbl)
        }
      }
      n96 = Absolute Value(x=w257) -> (abs(x)=w254:dbl)
      n97 = Absolute Value(x=w257) -> (abs(x)=w255:dbl)
      n98 = feedback #4(1000.0 ("Setpoint")) -> (w266:dbl)
      n99 = feedback-in #4(w265) -> ()
      n100 = feedback #5() -> (w263:i32)  [unwired: 1 in]
      n101 = Less?(x=w255, y=0.5) -> (x < y?=w258:bool)
      n102 = case shown="真" w258 {
        tunnel: w263 -> [_ w291]
        tunnel: [0 w289] -> w262
        frame False {
        }
        frame True {
          n103 = Add(x=w291, y=1) -> (x+y=w289:i32)
        }
      }
      n104 = feedback-in #5(w262) -> ()
      n105 = feedback #6() -> (w240:i32)  [unwired: 1 in]
      n106 = Less?(x=w254, y=0.2) -> (x < y?=w253:bool)
      n107 = case shown="真" w253 {
        tunnel: w240 -> [_ w295]
        tunnel: [0 w293] -> w264
        frame False {
        }
        frame True {
          n108 = Add(x=w295, y=1) -> (x+y=w293:i32)
        }
      }
      n109 = feedback-in #6(w264) -> ()
      n110 = Greater?(x=w263, y=w259) -> (0:w261:bool)
      n111 = Greater?(x=w240, y=w259) -> (0:w260:bool)
      n112 = Greater?(x=w270, y=0.0) -> (0:w247:bool)
      n113 = Greater?(x=0.0, y=w270) -> (0:w251:bool)
      n114 = case shown="假" w244 {
        tunnel: w240 -> [_ _]
        tunnel: w260 -> [w299 _]
        tunnel: w261 -> [w298 w308]
        tunnel: [w297 w307] -> w243
        tunnel: w247 -> [w296 w306]
        frame False {
          n115 = case shown="假" w299 {
            tunnel: [w301 w305] -> w297
            tunnel: w298 -> [w302 _]
            tunnel: w296 -> [w300 _]
            frame False {
              n116 = case shown="假" w302 {
                tunnel: [w303 w304] -> w301
                tunnel: w300 -> [_ _]
                frame False {
                  w303 = T6 4 items=["Unknow", "Stable", "Following Warm", "Following Cold", "Unfollowing"]
                }
                frame True {
                  w304 = T6 4 items=["Unknow", "Stable", "Following Warm", "Following Cold", "Unfollowing"]
                }
              }
            }
            frame True {
              w305 = T6 1 items=["Unknow", "Stable", "Following Warm", "Following Cold", "Unfollowing"]
            }
          }
        }
        frame True {
          n117 = case shown="假" w308 {
            tunnel: [w309 w310] -> w307
            tunnel: w306 -> [_ w311]
            frame False {
              w309 = T6 4 items=["Unknow", "Stable", "Following Warm", "Following Cold", "Unfollowing"]
            }
            frame True {
              n118 = case shown="真" w311 {
                tunnel: [w312 w313] -> w310
                frame False {
                  w312 = T6 3 items=["Unknow", "Stable", "Following Warm", "Following Cold", "Unfollowing"]
                }
                frame True {
                  w313 = T6 2 items=["Unknow", "Stable", "Following Warm", "Following Cold", "Unfollowing"]
                }
              }
            }
          }
        }
      }
      "下拉列表" <- w243
      n119 = feedback #7() -> (w241:i32)  [unwired: 1 in]
      n120 = case shown="假" w247 {
        tunnel: [0 w274] -> w248
        tunnel: w241 -> [_ w276]
        tunnel: w246 -> [_ w275]
        tunnel: [FALSE w273] -> _
        frame False {
        }
        frame True {
          n121 = Add(x=w276, y=1) -> (x+y=w274:i32)
          n122 = Greater?(x=w274, y=w275) -> (0:w273:bool)
        }
      }
      n123 = feedback-in #7(w248) -> ()
      n124 = feedback #8() -> (w249:i32)  [unwired: 1 in]
      n125 = case shown="假" w251 {
        tunnel: [0 w282] -> w250
        tunnel: w249 -> [_ w283]
        tunnel: w246 -> [_ w281]
        tunnel: [FALSE w280] -> _
        frame False {
        }
        frame True {
          n126 = Add(x=w283, y=1) -> (x+y=w282:i32)
          n127 = Greater?(x=w282, y=w281) -> (0:w280:bool)
        }
      }
      n128 = feedback-in #8(w250) -> ()
    }
  }
  n129 = flat-sequence "340-A cold head" {
    tunnel: w2 -> [w317]
    tunnel: w4 -> [w316]
    tunnel: w37 -> [w315]
    tunnel: [w314] -> w36
    frame #0 {
      w318 = 8 ("y")
      w332 = 5 ("y")
      n130 = Subtract(x=w317, y=w316) -> (x-y=w330:dbl)
      n131 = flat-sequence {
        tunnel: w316 -> [w361]
        tunnel: [w361] -> w339
        tunnel: w340 -> [w360]
        tunnel: [w359] -> w344
        frame #0 {
          n132 = Subtract(x=w361, y=w360) -> (x-y=w359:dbl)
        }
      }
      n133 = Absolute Value(x=w330) -> (abs(x)=w327:dbl)
      n134 = Absolute Value(x=w330) -> (abs(x)=w328:dbl)
      n135 = feedback #9(1000.0 ("Setpoint")) -> (w340:dbl)
      n136 = feedback-in #9(w339) -> ()
      n137 = feedback #10() -> (w336:i32)  [unwired: 1 in]
      n138 = Less?(x=w328, y=0.5) -> (x < y?=w331:bool)
      n139 = case shown="假" w331 {
        tunnel: w336 -> [_ w365]
        tunnel: [0 w363] -> w335
        frame False {
        }
        frame True {
          n140 = Add(x=w365, y=1) -> (x+y=w363:i32)
        }
      }
      n141 = feedback-in #10(w335) -> ()
      n142 = feedback #11() -> (w338:i32)  [unwired: 1 in]
      n143 = Less?(x=w327, y=0.2) -> (x < y?=w326:bool)
      n144 = case shown="真" w326 {
        tunnel: w338 -> [_ w369]
        tunnel: [0 w367] -> w337
        frame False {
        }
        frame True {
          n145 = Add(x=w369, y=1) -> (x+y=w367:i32)
        }
      }
      n146 = feedback-in #11(w337) -> ()
      n147 = Greater?(x=w336, y=w332) -> (0:w334:bool)
      n148 = Greater?(x=w338, y=w332) -> (0:w333:bool)
      n149 = Greater?(x=w344, y=0.0) -> (0:w319:bool)
      n150 = Greater?(x=0.0, y=w344) -> (0:w324:bool)
      n151 = case shown="假" w315 {
        tunnel: w338 -> [_ _]
        tunnel: w333 -> [w373 _]
        tunnel: w334 -> [w372 w382]
        tunnel: [w371 w381] -> w314
        tunnel: w319 -> [w370 w380]
        frame False {
          n152 = case shown="假" w373 {
            tunnel: [w375 w379] -> w371
            tunnel: w372 -> [w376 _]
            tunnel: w370 -> [w374 _]
            frame False {
              n153 = case shown="真" w376 {
                tunnel: [w377 w378] -> w375
                tunnel: w374 -> [_ _]
                frame False {
                  w377 = T6 4 items=["Unknow", "Stable", "Following Warm", "Following Cold", "Unfollowing"]
                }
                frame True {
                  w378 = T6 4 items=["Unknow", "Stable", "Following Warm", "Following Cold", "Unfollowing"]
                }
              }
            }
            frame True {
              w379 = T6 1 items=["Unknow", "Stable", "Following Warm", "Following Cold", "Unfollowing"]
            }
          }
        }
        frame True {
          n154 = case shown="假" w382 {
            tunnel: [w383 w384] -> w381
            tunnel: w380 -> [_ w385]
            frame False {
              w383 = T6 4 items=["Unknow", "Stable", "Following Warm", "Following Cold", "Unfollowing"]
            }
            frame True {
              n155 = case shown="真" w385 {
                tunnel: [w386 w387] -> w384
                frame False {
                  w386 = T6 3 items=["Unknow", "Stable", "Following Warm", "Following Cold", "Unfollowing"]
                }
                frame True {
                  w387 = T6 2 items=["Unknow", "Stable", "Following Warm", "Following Cold", "Unfollowing"]
                }
              }
            }
          }
        }
      }
      "下拉列表 2" <- w314
      n156 = feedback #12() -> (w321:i32)  [unwired: 1 in]
      n157 = case shown="假" w319 {
        tunnel: [0 w348] -> w320
        tunnel: w321 -> [_ w350]
        tunnel: w318 -> [_ w349]
        tunnel: [FALSE w347] -> _
        frame False {
        }
        frame True {
          n158 = Add(x=w350, y=1) -> (x+y=w348:i32)
          n159 = Greater?(x=w348, y=w349) -> (0:w347:bool)
        }
      }
      n160 = feedback-in #12(w320) -> ()
      n161 = feedback #13() -> (w322:i32)  [unwired: 1 in]
      n162 = case shown="真" w324 {
        tunnel: [0 w356] -> w323
        tunnel: w322 -> [_ w357]
        tunnel: w318 -> [_ w355]
        tunnel: [FALSE w354] -> _
        frame False {
        }
        frame True {
          n163 = Add(x=w357, y=1) -> (x+y=w356:i32)
          n164 = Greater?(x=w356, y=w355) -> (0:w354:bool)
        }
      }
      n165 = feedback-in #13(w323) -> ()
    }
  }
  n166 = Bundle("Kelvin Reading"=w1, "Setpoint"=w3, "Heater Range 340-Loop2"=w22, "Output Value"=w25, "Ramping Active/Inactive"=w26, w39, "Kelvin Reading"=w2, "Setpoint"=w4, "Heater Range"=w38, "Heater Output"=w41, "Ramping Active/Inactive"=w37, w36, FALSE) -> (→"output":T8)  [unwired: 1 in]
  "Output Field (Gs)" <- w14
